vi "AMWave.vi"() -> ()   [LabVIEW 2014]
uses:
  <vilib>/imath/engines/lvmath2/RunTimeEngine/Managers/WorkSpace/UID Generator.vi
  <vilib>/imath/engines/lvmath2/RunTimeEngine/RunTimeType/NIMS_RunTimeType_From StrictType (excl LVString).vi
  <instcachedir>/0/NIMS_RunTimeType_From StrictType (excl LVString)_6F30FCEAD152B34FB6BC3D48AAFE00E6.lvgen/NIMS_RunTimeType_From StrictType (excl LVString)_6F30FCEAD152B34FB6BC3D48AAFE00E6_000.vi
  <vilib>/imath/engines/lvmath2/RunTimeEngine/LocalVariableDefStatement/MC_LocalVariableDefStatement_Display.vi
  <vilib>/imath/engines/lvmath2/RunTimeEngine/RangeToken/NIMS_Range.vi
  <instcachedir>/0/NIMS_Range_6DDDFF7386AB584A9063FA25EAF603C1.lvgen/NIMS_Range_6DDDFF7386AB584A9063FA25EAF603C1_000.vi
  <vilib>/imathl/engines/lvmath/Functions/Error Handling/Create Error.vi
  <vilib>/imath/engines/lvmath2/RunTimeEngine/ArithmeticOperatorToken/NIMS_ArithmeticOperator_times.vi
  <instcachedir>/0/NIMS_ArithmeticOperator_times_831F30C6BFCCF94698B6F46369084E97.lvgen/NIMS_ArithmeticOperator_times_831F30C6BFCCF94698B6F46369084E97_000.vi
  <vilib>/imath/engines/lvmath2/RunTimeEngine/Managers/SymbolTable/Clear UID.vi
  <vilib>/imath/engines/lvmath2/RunTimeEngine/NodeEndStatement/NIMS_NodeEndStatement_Output.vi
  <instcachedir>/0/NIMS_NodeEndStatement_Output_53EC0D466D134D7ABD903AC30B43404B.lvgen/NIMS_NodeEndStatement_Output_53EC0D466D134D7ABD903AC30B43404B_005.vi
  <vilib>/imath/engines/lvmath2/RunTimeEngine/ErrorHandling/NIMS_Finalize Error.vi
  <vilib>/imath/engines/lvmath2/RunTimeEngine/Managers/SymbolTable/NIMS_WorkSpace.lvlib
panel:
  in  "Waveform Parameters":T1
  in  "Digitizing Parameters":T2
  out "Displacement":dbl[](array[numeric])
  out "Time":dbl[](array[numeric])
  out "XY Graph":cluster{"t":dbl[], "x":dbl[]}(graph)
  # "Parameters controlling\nwaveform  signal\nsampling"
  # "X and Y var. indicators"
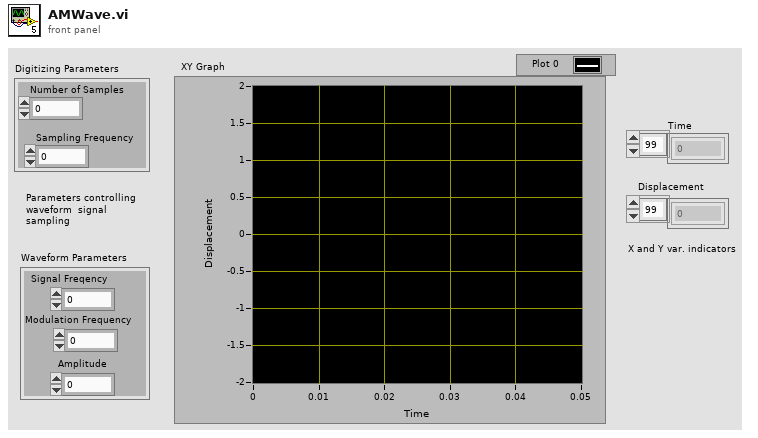
[diagram p1: front panel]
types:
  T1 = cluster{"Signal Freqency":dbl, "Modulation Frequency":dbl, "Amplitude":dbl}
  T2 = cluster{"Number of Samples":dbl, "Sampling Frequency":dbl}
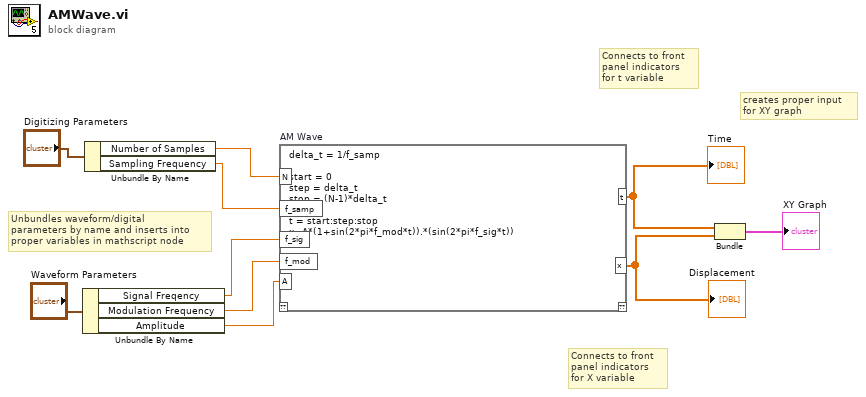
[diagram p0: block diagram]
diagram:
  # "Connects to front\npanel indicators\nfor t variable"
  # "Connects to front\npanel indicators \nfor X variable"
  # "creates proper input \nfor XY graph"
  # "Creates time vector via digitizing parameters\nand plugs into function for amplitude \nmodulated wave, containing waveform parameters"
  # "Unbundles waveform/digital\nparameters by name and inserts into \nproper variables in mathscript node"
  n1 = Unbundle By Name("Waveform Parameters") -> ("Signal Freqency"=w5:dbl, "Modulation Frequency"=w4:dbl, "Amplitude"=w3:dbl)
  n2 = Unbundle By Name("Digitizing Parameters") -> ("Number of Samples"=w8:dbl, "Sampling Frequency"=w7:dbl)
  n3 = mathscript code="delta_t = 1/f_samp\n\nstart = 0\nstep = delta_t\nstop = (N-1)*delta_t\n\nt = start:step:stop\nx=A*(1+sin(2*pi*f_mod*t)).*(sin(2*pi*f_sig*t))" "AM Wave"("f_samp"=w7, "f_sig"=w5, "A"=w3, "N"=w8, "f_mod"=w4) -> ("x"=w2:dbl[], "t"=w1:dbl[])  [unwired: 1 in, 1 out]
  "Time" <- w1
  "Displacement" <- w2
  n4 = Bundle("t"=w1, "x"=w2) -> (→"XY Graph":cluster{"t":dbl[], "x":dbl[]})  [unwired: 1 in]
